vi "Launcher - MainUI.vi"(6 "Worker Alias":string="MainUI", 8 "error in":errorcluster, 9 "Initialization Data":T1, 11 "MainUI in":refnum<class "MainUI.lvclass">) -> (0 "error out":errorcluster)   [LabVIEW 2024]
doc: "This VI launches the Head Worker of a Workers application."
uses:
  Workers/MainUI/Initialization Data.ctl
  Workers/MainUI/Response Cases.ctl
  Workers/MainUI/MainUI.lvclass
  C:/Program Files (x86)/National Instruments/LabVIEW 2024/vi.lib/addons/_Workers/Library/Classes/Worker/Worker.lvclass
  <vilib>/addons/_Workers/Debugger/Debug Client/Debug Client.lvlib
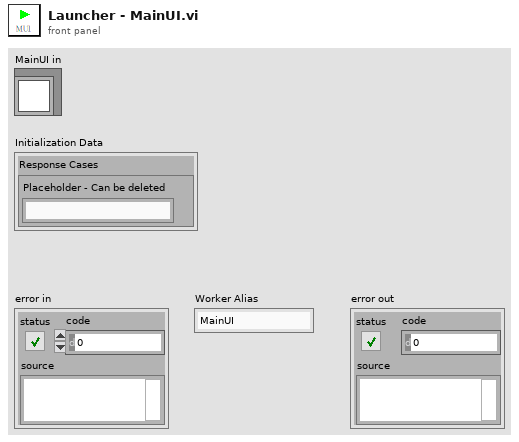
[diagram p1: front panel]
types:
  T1 = typedef "MainUI.lvclass/Initialization Data.ctl" = cluster{"Response Cases":T2}
  T2 = typedef "MainUI.lvclass/Response Cases.ctl" = cluster{"Placeholder - Can be deleted":string}
  T3 = enum32{"Invalid", "Standard", "Closed", "Hidden", "Minimized", "Maximized"}
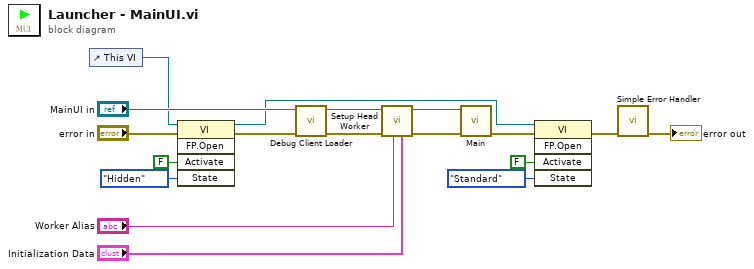
[diagram p0: block diagram]
diagram:
  n1 = control-ref of="This VI"() -> (w8:refnum<vi>)
  n2 = invoke class="VI" method="FP.Open"(reference=w8, error in="error in", "Activate"=FALSE ("Activate?"), "State"=T3."Hidden") -> (reference out=w3:refnum<vi>, error out=w9:errorcluster)  [unwired: 1 in, 3 out]
  n3 = call <vilib>:"Debug Client Loader.vi"("error in (no error)"=w9, "Worker_"="MainUI in") -> ("error out"=w12:errorcluster, "Worker_out"=w10:refnum<class "MainUI.lvclass">)  [unwired: 8 in]
  n4 = call-dynamic "Setup Head Worker.vi"("Initalization Data"="Initialization Data", "Worker Alias"="Worker Alias", "error in"=w12, "Worker_"=w10) -> ("error out"=w18:errorcluster, "Worker_out"=w16:refnum<class "MainUI.lvclass">)  [unwired: 6 in]
  n5 = call-dynamic "Main.vi"("error in"=w18, "MainUI in"=w16) -> ("error out"=w2:errorcluster)  [unwired: 8 in, 1 out]
  n6 = invoke class="VI" method="FP.Open"(reference=w3, error in=w2, "Activate"=FALSE ("Activate?"), "State"=T3."Standard") -> (error out=w1:errorcluster)  [unwired: 1 in, 4 out]
  n7 = call <vilib>:"Simple Error Handler.vi"("error in (no error)"=w1) -> ("error out"=→"error out":errorcluster)  [unwired: 4 in, 4 out]
